vi "CheckEquiments.vi"(0 "reference in":refnum<class "Test.lvclass">, 5 "error in (no error)":errorcluster) -> (14 "reference out":refnum<class "Test.lvclass">, 19 "error out":errorcluster)   [LabVIEW 2024, in "Test.lvclass"]
uses:
  Test.lvclass
  Test.lvclass/Test.ctl
panel:
  # "Connector Pane"
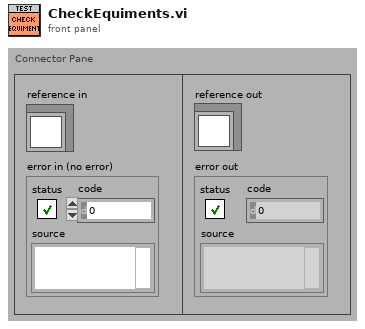
[diagram p1: front panel]
types:
  T1 = typedef "Test.lvclass/ObjectAttributes.ctl" = cluster{"Engine":bool, "Dynamometer":bool, "Test Status":enum16{"Test Start", "Test Continue", "Test Failed", "Test Success"}, "History String":string}
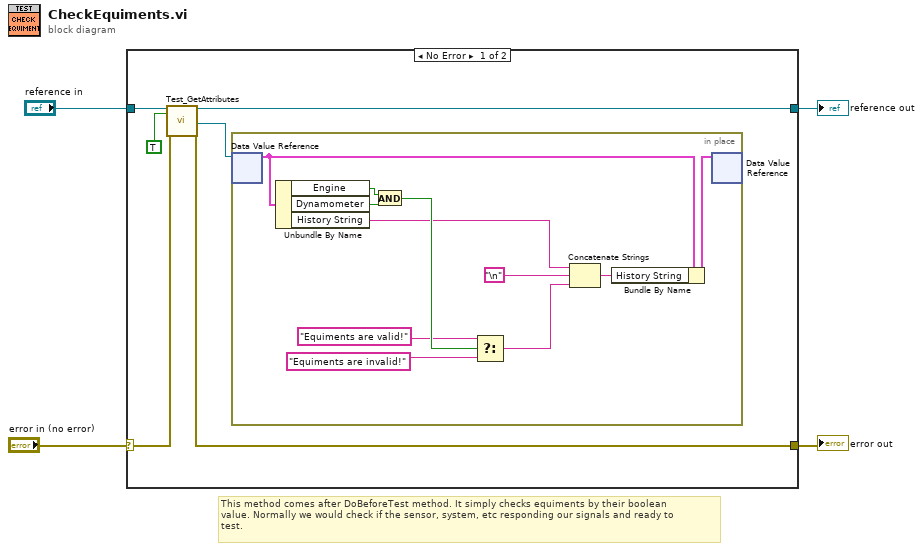
[diagram p0: block diagram]
diagram:
  # "This method comes after DoBeforeTest method. It simply checks equiments by their boolean\nvalue. Normally we would check if the sensor, system, etc responding our signals and ready to \ntest."
  n1 = case shown="No Error" "error in (no error)" {
    selector: "error in (no error)" -> [w10 w23]
    tunnel: [w9 w23] -> w3
    tunnel: [w7 w22] -> w1
    tunnel: "reference in" -> [w8 w22]
    frame No Error {
      n2 = call "Test_GetAttributes.vi"("reference in"=w8, "OnlyGetDvrReference(False)"=TRUE, "error in (no error)"=w10) -> ("reference out"=w7:refnum<class "Test.lvclass">, "DataRef"=w6:refnum<data-value>, "error out"=w9:errorcluster)  [unwired: 13 in, 1 out]
      n3 = in-place {
        n4 = in-place-dvr #1(w6) -> (w18:T1)  [unwired: 1 out]
        n5 = Unbundle By Name(w18) -> ("Engine"=w17:bool, "Dynamometer"=w16:bool, "History String"=w13:string)
        n6 = And(x=w17, y=w16) -> (x .and. y?=w21:bool)
        n7 = Select(t="Equiments are valid!", s=w21, f="Equiments are invalid!") -> (s? t:f=w12:string)
        n8 = Concatenate Strings(w13, "\n", w12) -> (w14:string)
        n9 = Bundle By Name(cluster=w18, "History String"=w14) -> (w15:T1)
        n10 = in-place-dvr #1(w15) -> ()  [unwired: 2 out]
      }
    }
    frame Error {
    }
  }
  "error out" <- w3
  "reference out" <- w1
